vi "Continuous Moments.vi"   [LabVIEW 2020, in "NI_Gmath.lvlib"]
doc: "Returns the expected mean and variance of the random variate X, where X describes the selected distribution type. You must manually select the polymorphic instance to use."
uses:
  <vilib>/gmath/NI_Gmath.lvlib
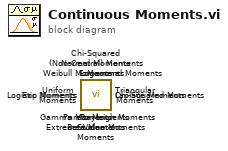
[diagram p0: block diagram]
diagram:
  n1 = call <vilib>:"Pareto Moments.vi"() -> ()  [unwired: 9 in, 3 out]
  n2 = call <vilib>:"Lognormal Moments.vi"() -> ()  [unwired: 9 in, 3 out]
  n3 = call <vilib>:"Logistic Moments.vi"() -> ()  [unwired: 9 in, 3 out]
  n4 = call <vilib>:"Laplace Moments.vi"() -> ()  [unwired: 9 in, 3 out]
  n5 = call <vilib>:"Extreme Value Moments.vi"() -> ()  [unwired: 9 in, 3 out]
  n6 = call <vilib>:"Chi-Squared (Non-Central) Moments.vi"() -> ()  [unwired: 9 in, 3 out]
  n7 = call <vilib>:"Weibull Moments.vi"() -> ()  [unwired: 9 in, 3 out]
  n8 = call <vilib>:"Uniform Moments.vi"() -> ()  [unwired: 9 in, 3 out]
  n9 = call <vilib>:"Triangular Moments.vi"() -> ()  [unwired: 9 in, 3 out]
  n10 = call <vilib>:"Student t Moments.vi"() -> ()  [unwired: 9 in, 3 out]
  n11 = call <vilib>:"Rayleigh Moments.vi"() -> ()  [unwired: 9 in, 3 out]
  n12 = call <vilib>:"Normal Moments.vi"() -> ()  [unwired: 9 in, 3 out]
  n13 = call <vilib>:"F Moments.vi"() -> ()  [unwired: 9 in, 3 out]
  n14 = call <vilib>:"Gamma Moments.vi"() -> ()  [unwired: 9 in, 3 out]
  n15 = call <vilib>:"Exp Moments.vi"() -> ()  [unwired: 9 in, 3 out]
  n16 = call <vilib>:"Chi-Squared Moments.vi"() -> ()  [unwired: 9 in, 3 out]
  n17 = call <vilib>:"Beta Moments.vi"() -> ()  [unwired: 9 in, 3 out]
